vi "Actor Core.vi"(8 "error in":errorcluster, 11 "TimerSensor in":refnum<class "TimerSensor.lvclass">) -> (0 "error out":errorcluster, 3 "Actor out":refnum<class "Actor.lvclass">)   [LabVIEW 2012, in "TimerSensor.lvlib" / "TimerSensor.lvclass"]
doc: "(<B>Filename</B>: Actor Framework.lvlib:Actor.lvclass:Actor Core.vi)\n\nReceives messages to the actor, reacts to them, and initiates any error handling that may shut the actor down.\n\nDescendant classes may override this VI to append parallel tasks for the actor to complete while it handles messages. Overrides use the Call Parent Method node."
uses:
  TimerSensor.lvclass
  <vilib>/ActorFramework/Actor/Actor.lvclass
  TimerViewSmall.lvclass
  TimerViewDetail.lvclass
  TimerSensorCharm.lvclass
  Sensor Definition/Sensor.lvclass/Sensor.ctl
  Sensor Definition/Sensor.lvclass
  Sensor Definition/Sensor/Write SmallView Actor.vi
  Sensor Definition/Sensor/Write DetailedView Actor.vi
  Sensor Definition/Sensor/Write CharmView Actor.vi
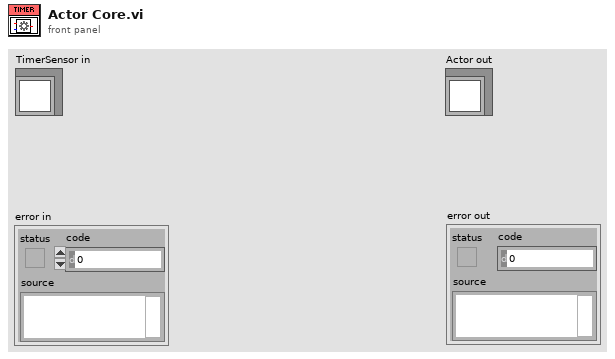
[diagram p1: front panel]
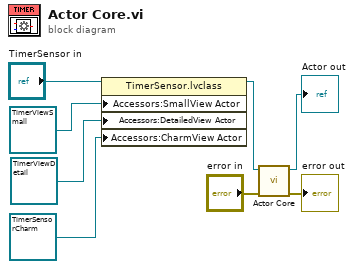
[diagram p0: block diagram]
diagram:
  n1 = property class="TimerSensor.lvclass"(reference="TimerSensor in", "Accessors:SmallView Actor"=refnum<class "TimerViewSmall.lvclass"> refnum ("TimerSensor.lvlib:TimerViewSmall.lvclass"), "Accessors:DetailedView Actor"=refnum<class "TimerViewDetail.lvclass"> refnum ("TimerSensor.lvlib:TimerViewDetail.lvclass"), "Accessors:CharmView Actor"=refnum<class "TimerSensorCharm.lvclass"> refnum ("TimerSensor.lvlib:TimerSensorCharm.lvclass")) -> (reference out=w4:refnum<class "TimerSensor.lvclass">)  [unwired: 1 in, 1 out]
  n2 = call-parent "Actor Core.vi"("error in"="error in", "Sensor in"=w4) -> ("error out"=→"error out":errorcluster, "Actor out"=→"Actor out":refnum<class "Actor.lvclass">)  [unwired: 8 in]
